vi "CS_Initialize_multiple.vi"() -> ()   [LabVIEW 2013, in "LightField Automation.lvclass"]
uses:
  LightField Automation.lvclass
  CS_LFAClassGlobal.vi
panel:
  in  "Instances":i32=2
  in  "stop":bool
  in  "Is Visible?":bool=TRUE
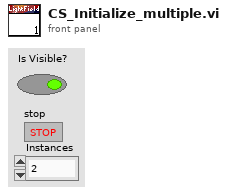
[diagram p1: front panel]
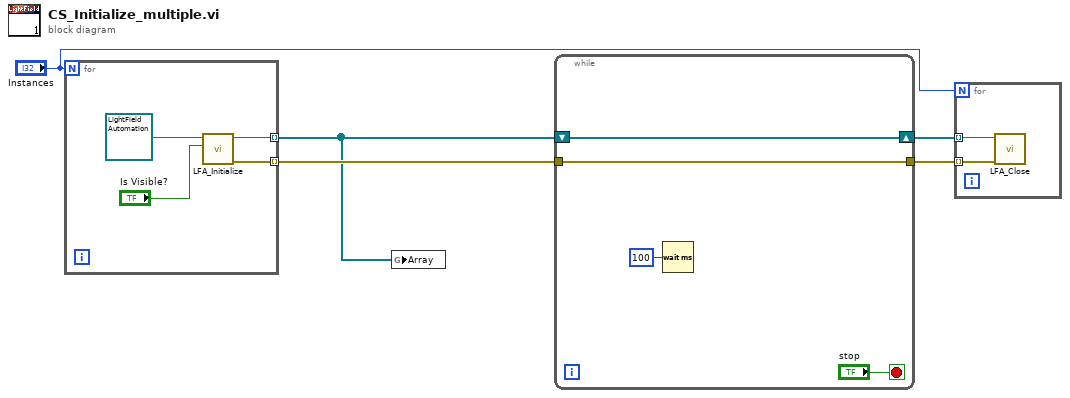
[diagram p0: block diagram]
diagram:
  n1 = for {
    N: "Instances" -> [_]
    tunnel: [w7] -> w2 mode=indexing
    tunnel: [w6] -> w4 mode=indexing
    n2 = call "LFA_Initialize.vi"("Is Visible?"="Is Visible?", "LightField Automation in"=refnum<class "LightField Automation.lvclass"> refnum ("LightField Automation.lvclass")) -> ("error out"=w6:errorcluster, "LightField Automation out"=w7:refnum<class "LightField Automation.lvclass">)  [unwired: 8 in]
  }
  n3 = global write "CS_LFAClassGlobal.vi" "Array"(w2) -> ()
  n4 = while {
    shift-right: [w12] -> w5
    shift-left: w2 -> [w12]
    tunnel: w4 -> [w11]
    tunnel: [w11] -> w3
    stop <- "stop" stop-if-true
    n5 = Wait (ms)(milliseconds to wait=u32 100) -> ()  [unwired: 1 out]
  }
  n6 = for {
    N: "Instances" -> [_]
    tunnel: w5 -> [w15] mode=indexing
    tunnel: w3 -> [w14] mode=indexing
    n7 = call "LFA_Close.vi"("error in (no error)"=w14, "LightField Automation in"=w15) -> ()  [unwired: 8 in, 2 out]
  }
